vi "Error Message.vi"(8 "error in (no error)":errorcluster {"code" format="%.0x"}, 10 "error code":i32 format="%.0g", 11 "instrument handle":refnum<k15>) -> (0 "error out":errorcluster {"code" format="%.0x"}, 2 "error message":string, 3 "instrument handle out":refnum<k15>)   [LabVIEW 2009, in "Keysight XSAn.lvlib"]
doc: "Translates the error return value from an IVI driver VI to a user-readable string. The user should pass a buffer with at least 256 bytes for the ErrorMessage parameter."
uses:
  <instrlib>/Keysight XSAn/Keysight XSAn.lvlib
  AgXSAn.dll
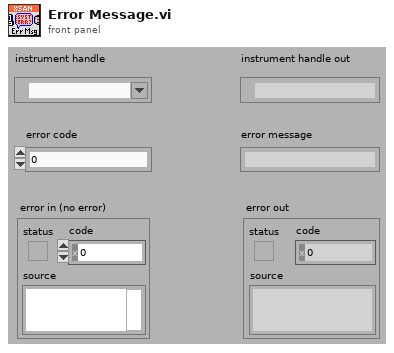
[diagram p1: front panel]
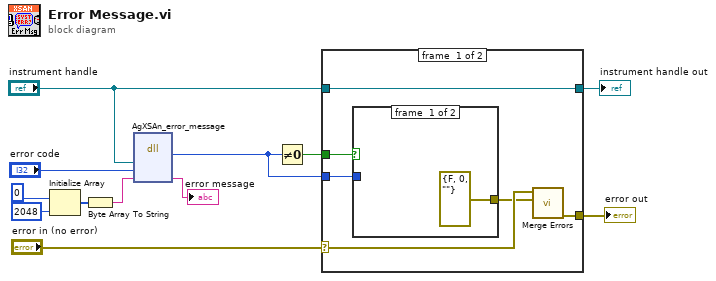
[diagram p0: block diagram]
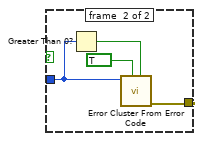
[diagram p2: hidden frame]
diagram:
  n1 = Initialize Array(u8 0, 2048 ("size of error message")) -> (w11:u8[])
  n2 = Byte Array To String(unsigned byte array=w11) -> (string=w9:string)
  n3 = dll-call lib="AgXSAn**.dll" fn="AgXSAn_error_message" ("LabVIEW:IviSpecAn_error_message")("instrument handle"="instrument handle", "error code"="error code", "error message"=w9) -> ("Status"=w4:i32, "error message"=→"error message":string)  [unwired: 4 in, 3 out]
  n4 = Not Equal To 0?(x=w4) -> (x != 0?=w6:bool)
  n5 = case shown="No Error" "error in (no error)" {
    selector: "error in (no error)" -> [w16 w25]
    tunnel: [w14 w25] -> w3
    tunnel: w6 -> [w18 _]
    tunnel: w4 -> [w17 _]
    tunnel: "instrument handle" -> [w13 w24]
    tunnel: [w13 w24] -> w1
    frame #0 {
      n6 = case shown="True" w18 {
        tunnel: [errorcluster {"status"=FALSE, "code"=0, "source"=""} ("error out") w21] -> w15
        tunnel: w17 -> [_ w20]
        frame #0 {
        }
        frame #1 {
          n7 = Greater Than 0?(x=w20) -> (x > 0?=w22:bool)
          n8 = call <vilib>:"Error Cluster From Error Code.vi"("is warning? (False)"=w22, "show call chain? (False)"=TRUE, "error code (0)"=w20) -> ("error out"=w21:errorcluster)  [unwired: 1 in, 5 out]
        }
      }
      n9 = call <vilib>:"Merge Errors.vi"("error in 2 (no error)"=w15, "error in 1 (no error)"=w16) -> ("error out"=w14:errorcluster)  [unwired: 2 in, 3 out]
    }
    frame #1 {
    }
  }
  "instrument handle out" <- w1
  "error out" <- w3
